vi "Dbl Array_Slice.vi"(8 "Error":errorcluster, 9 "End Index\n(-1) Last point":i32, 10 "Start Index":i32, 11 "Array":dbl[](array[numeric]) format="%.2f") -> (0 "Error Out":errorcluster, 1 "End Out":i32, 2 "Start Out":i32, 3 "Subarray (array[i:j]) Out":dbl[](array[numeric]) format="%.2f")   [LabVIEW 2025]
doc: "Returns a subset from <B>array</B>. <B>subset</B> has the following syntax:\n\narray[subset] = subarray\n\nsubset is a range and is of the form \"i:j\" where i and j are integers\nif i is ommitted it is assumed to be zero. If j is ommitted it is assumed to be length(array)\nif i or j are negative numbers they are assumed to be refferenced from the end of the string.\nexamples:\n\nif array = [7,6,5,4,3,2,1]\n\nstring[2:] = [5,4,3,2,1]\nstring[:3] = [7,6,5]\nstring[-1] = [1]\nstring[4] = [3]\nstring[-4:-2] = [4,3]"
panel:
  # "Slice 1D Array.vi\n\nReturns a subset from array\n\nPlease visit http://www.OpenG.org to learn about the\nOpen Source LabVIEW software movement.\n\nNOTICE -- YOU MUST LEAVE THIS NOTICE IN PLACE.  PER THE TERMS OF THE LICENSE BELOW, YOU MAY SUBLICENSE THIS SOFTWARE \nIN ANY WAY THAT DOES NOT CONFLICT WITH THIS LICENSE.\n\n### BSD License (http://www.opensource.org/licenses/bsd-license.php) Begin ###\n \nCopyright (c) 2002, Jim Kring <jim@jimkring.com>\nCopyright (c) 2002, Cal-Bay Systems, Inc. <info@calbay.com>\n\nAll rights reserved.\n\nRedistribution and use in source and binary forms, with or without modification, are permitted provided that the following conditions are met:\n\n    * Redistributions of source code must retain the above copyright notice, this list of conditions and the following disclaimer.\n    * Redistributions in binary form must reproduce the above copyright notice, this list of conditions and the following disclaimer in the \n       documentation and/or other materials provided with the distribution.\n    * Neither the name of SciWare, James Kring, Inc., nor the names of its contributors may be used to endorse or promote products derived \n       from this software without specific prior written permission.\n\nTHIS SOFTWARE IS PROVIDED BY THE COPYRIGHT HOLDERS AND CONTRIBUTORS \"AS IS\" AND ANY EXPRESS OR IMPLIED WARRANTIES, \nINCLUDING, BUT NOT LIMITED TO, THE IMPLIED WARRANTIES OF MERCHANTABILITY AND FITNESS FOR A PARTICULAR PURPOSE ARE \nDISCLAIMED. IN NO EVENT SHALL THE COPYRIGHT OWNER OR CONTRIBUTORS BE LIABLE FOR ANY DIRECT, INDIRECT, INCIDENTAL,\n SPECIAL, EXEMPLARY, OR CONSEQUENTIAL DAMAGES (INCLUDING, BUT NOT LIMITED TO, PROCUREMENT OF SUBSTITUTE GOODS OR \nSERVICES; LOSS OF USE, DATA, OR PROFITS; OR BUSINESS INTERRUPTION) HOWEVER CAUSED AND ON ANY THEORY OF LIABILITY, \nWHETHER IN CONTRACT, STRICT LIABILITY, OR TORT (INCLUDING NEGLIGENCE OR OTHERWISE) ARISING IN ANY WAY OUT OF THE USE \nOF THIS SOFTWARE, EVEN IF ADVISED OF THE POSSIBILITY OF SUCH DAMAGE.\n\n### BSD License End ###"
  # "[OpenG VI Tags] ***Do Not Remove***\nSVN Revision = 593\nSVN Revision Date = 2007-01-18 16:52:28 -0800 (Thu, 18 Jan 2007)\nPackage = oglib_array-2.7-1\nDepends = oglib_string-2.6-1"
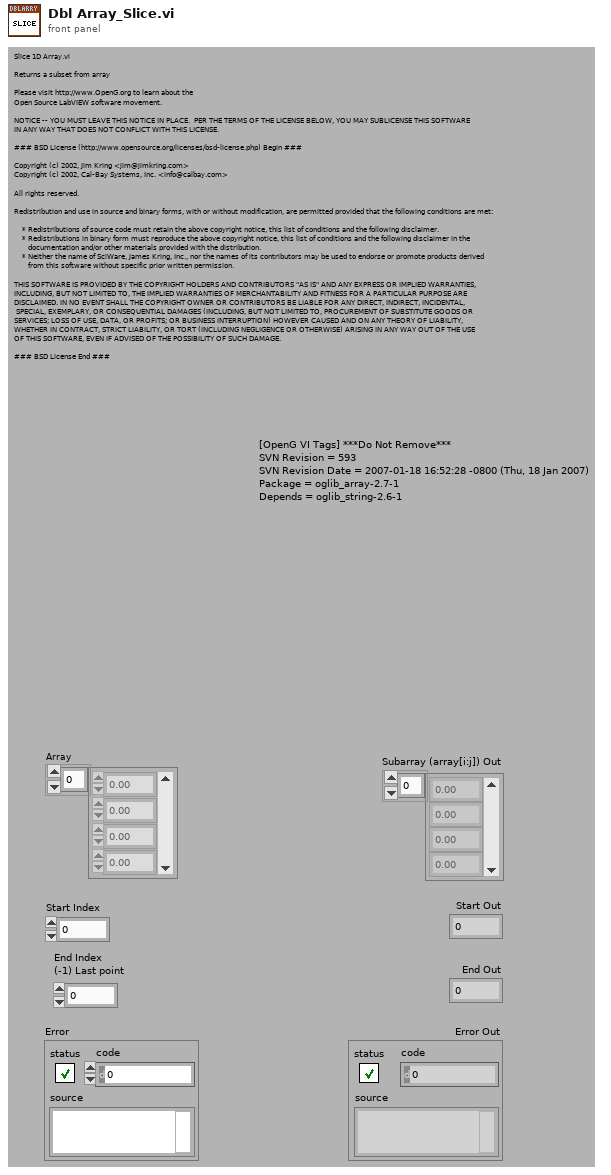
[diagram p1: front panel]
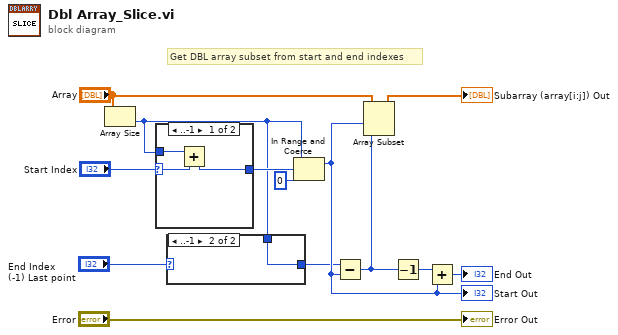
[diagram p0: block diagram]
diagram:
  # "Get DBL array subset from start and end indexes"
  n1 = Array Size(array="Array") -> (size(s)=w1:i32)
  n2 = case shown="..-1" "Start Index" {
    selector: "Start Index" -> [w15 w17]
    tunnel: [w14 w17] -> w2
    tunnel: w1 -> [w16 _]
    frame ..-1 {
      n3 = Add(x=w16, y=w15) -> (x+y=w14:i32)
    }
    frame 0.. {
    }
  }
  n4 = case shown="..-1" "End Index\n(-1) Last point" {
    selector: "End Index\n(-1) Last point" -> [w18 _]
    tunnel: w1 -> [_ w19]
    tunnel: [w18 w19] -> w4
    frame 0.. {
    }
    frame ..-1 {
    }
  }
  n5 = In Range and Coerce(upper limit=w1, x=w2, lower limit=0 ("upper limit")) -> (coerced(x)=w7:i32)  [unwired: 1 out]
  "Start Out" <- w7
  n6 = Subtract(x=w4, y=w7) -> (x-y=w12:i32)
  n7 = Array Subset(array="Array", index=w7, length=w12) -> (→"Subarray (array[i:j]) Out":dbl[])
  n8 = Decrement(x=w12) -> (x-1=w11:i32)
  n9 = Add(x=w11, y=w7) -> (x+y=→"End Out":i32)
  "Error Out" <- "Error"
